vi "Angle_Step.vi"   [LabVIEW 2018]
uses:
  Global/Global Variables/global.vi
  Instrument_Setup.vi
  Global/Global Variables/Data_Display_global.vi
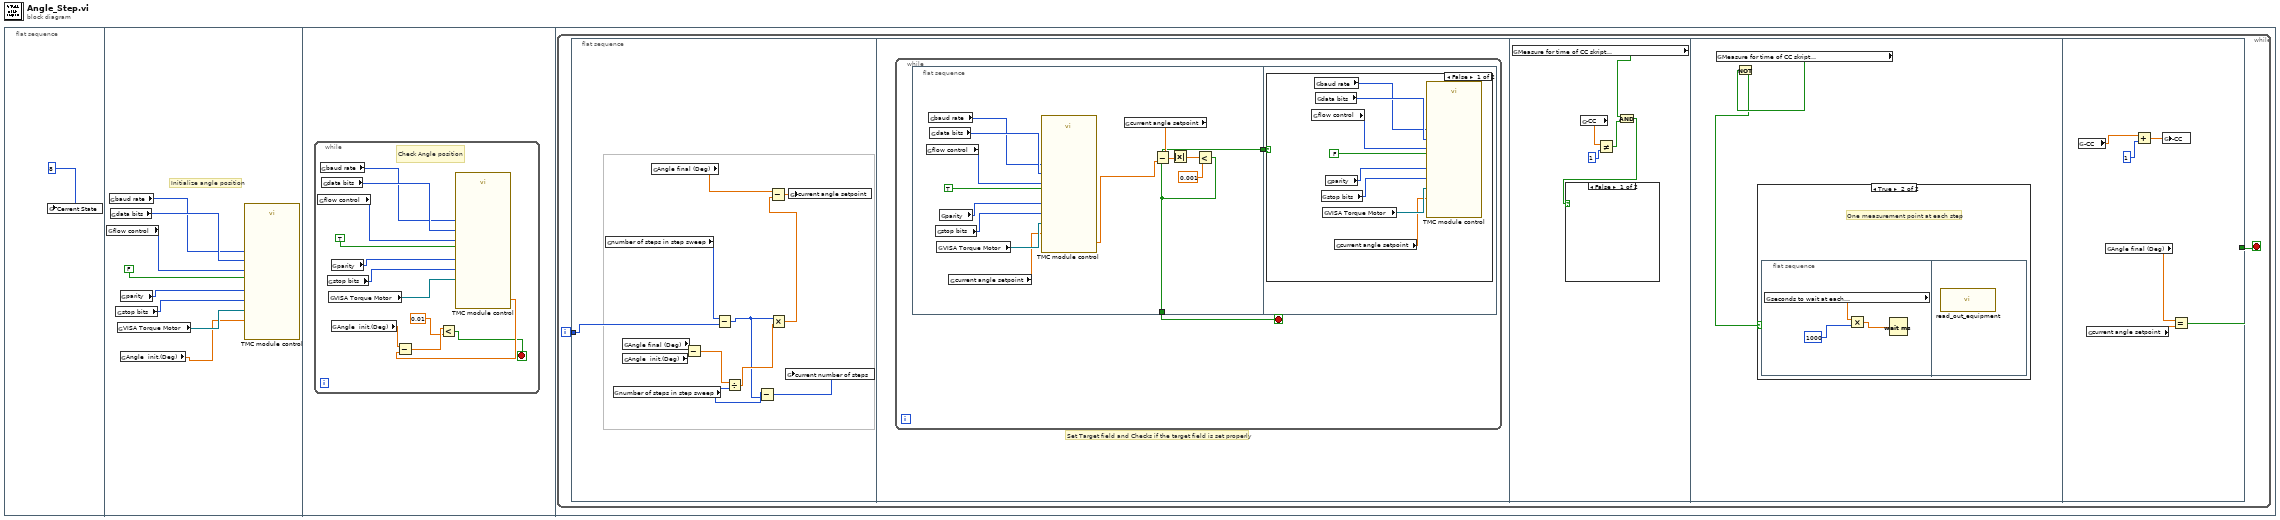
[diagram p0: block diagram]
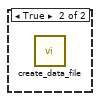
[diagram p3: hidden frame]
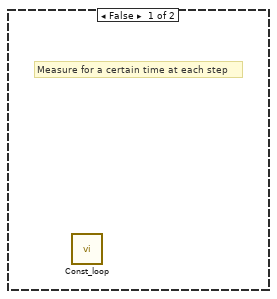
[diagram p4: hidden frame]
diagram:
  n1 = flat-sequence {
    frame #0 {
      n2 = global write "global.vi" "Cerrent State"(8) -> ()
    }
    frame #1 {
      # "Initialize angle position"
      n3 = global read "Instrument_Setup.vi" "flow control"() -> (w9:u16)
      n4 = global read "Instrument_Setup.vi" "baud rate"() -> (w7:u32)
      n5 = global read "Instrument_Setup.vi" "data bits"() -> (w8:u16)
      n6 = global read "Instrument_Setup.vi" "stop bits"() -> (w5:u16)
      n7 = global read "Instrument_Setup.vi" "VISA Torque Motor"() -> (w3:refnum<visa-resource-name>)
      n8 = global read "Instrument_Setup.vi" "parity"() -> (w6:u16)
      n9 = global read "global.vi" "Angle  init.(Deg)"() -> (w2:dbl)
      n10 = call "TMC module control.vi"("Nur Position auslesen"=FALSE, "Winkel [°]"=w2, "flow control"=w9, "VISA resource name"=w3, "stop bits"=w5, "parity"=w6, "data bits"=w8, "baud rate"=w7) -> ()  [unwired: 2 out]
    }
    frame #2 {
      n11 = while {
        stop <- w10 stop-if-true
        # "Check Angle position"
        n12 = global read "Instrument_Setup.vi" "flow control"() -> (w21:u16)
        n13 = global read "Instrument_Setup.vi" "baud rate"() -> (w19:u32)
        n14 = global read "Instrument_Setup.vi" "data bits"() -> (w20:u16)
        n15 = global read "Instrument_Setup.vi" "stop bits"() -> (w17:u16)
        n16 = global read "Instrument_Setup.vi" "VISA Torque Motor"() -> (w15:refnum<visa-resource-name>)
        n17 = global read "Instrument_Setup.vi" "parity"() -> (w18:u16)
        n18 = global read "global.vi" "Angle  init.(Deg)"() -> (w14:dbl)
        n19 = call "TMC module control.vi"("Nur Position auslesen"=TRUE, "flow control"=w21, "VISA resource name"=w15, "stop bits"=w17, "parity"=w18, "data bits"=w20, "baud rate"=w19) -> ("Ausgelesener Winkel [°]"=w13:dbl)  [unwired: 1 in, 1 out]
        n20 = Subtract(x=w14, y=w13) -> (x-y=w12:dbl)
        n21 = Less?(x=w12, y=0.01) -> (x < y?=w10:bool)
      }
    }
    frame #3 {
      n22 = while {
        i -> [w22]
        stop <- w23 stop-if-true
        n23 = flat-sequence {
          tunnel: w22 -> [w24]
          tunnel: [w75] -> w23
          frame #0 {
            n24 = global read "global.vi" "number of steps in step sweep"() -> (w31:i32)
            n25 = global read "global.vi" "number of steps in step sweep"() -> (w29:i32)
            n26 = global read "global.vi" "Angle final (Deg)"() -> (w27:dbl)
            n27 = global read "global.vi" "Angle  init.(Deg)"() -> (w26:dbl)
            n28 = global read "global.vi" "Angle final (Deg)"() -> (w35:dbl)
            n29 = Subtract(x=w27, y=w26) -> (x-y=w25:dbl)
            n30 = Subtract(x=w31, y=w24) -> (x-y=w28:i32)
            n31 = Divide(x=w25, y=w29) -> (x/y=w33:dbl)
            n32 = Subtract(x=w29, y=w28) -> (x-y=w30:i32)
            n33 = Multiply(x=w28, y=w33) -> (x*y=w34:dbl)
            n34 = Subtract(x=w35, y=w34) -> (x-y=w32:dbl)
            n35 = global write "Data_Display_global.vi" "current number of steps"(w30) -> ()
            n36 = global write "Data_Display_global.vi" "current angle setpoint"(w32) -> ()
          }
          frame #1 {
            # "Set Target field and Checks if the target field is set properly"
            n37 = while {
              stop <- w36 stop-if-true
              n38 = flat-sequence {
                tunnel: [w47] -> w37
                tunnel: [w47] -> w36
                tunnel: w37 -> [w52]
                frame #0 {
                  n39 = global read "Instrument_Setup.vi" "flow control"() -> (w45:u16)
                  n40 = global read "Instrument_Setup.vi" "baud rate"() -> (w43:u32)
                  n41 = global read "Instrument_Setup.vi" "data bits"() -> (w44:u16)
                  n42 = global read "Instrument_Setup.vi" "stop bits"() -> (w41:u16)
                  n43 = global read "Instrument_Setup.vi" "VISA Torque Motor"() -> (w39:refnum<visa-resource-name>)
                  n44 = global read "Instrument_Setup.vi" "parity"() -> (w42:u16)
                  n45 = global read "Data_Display_global.vi" "current angle setpoint"() -> (w38:dbl)
                  n46 = call "TMC module control.vi"("Nur Position auslesen"=TRUE, "Winkel [°]"=w38, "flow control"=w45, "VISA resource name"=w39, "stop bits"=w41, "parity"=w42, "data bits"=w44, "baud rate"=w43) -> ("Ausgelesener Winkel [°]"=w46:dbl)  [unwired: 1 out]
                  n47 = global read "Data_Display_global.vi" "current angle setpoint"() -> (w48:dbl)
                  n48 = Subtract(x=w48, y=w46) -> (x-y=w50:dbl)
                  n49 = Absolute Value(x=w50) -> (abs(x)=w49:dbl)
                  n50 = Less?(x=w49, y=0.001) -> (x < y?=w47:bool)
                }
                frame #1 {
                  n51 = case shown="False" w52 {
                    frame False {
                      n52 = global read "Instrument_Setup.vi" "flow control"() -> (w60:u16)
                      n53 = global read "Instrument_Setup.vi" "baud rate"() -> (w58:u32)
                      n54 = global read "Instrument_Setup.vi" "data bits"() -> (w59:u16)
                      n55 = global read "Instrument_Setup.vi" "stop bits"() -> (w56:u16)
                      n56 = global read "Instrument_Setup.vi" "VISA Torque Motor"() -> (w54:refnum<visa-resource-name>)
                      n57 = global read "Instrument_Setup.vi" "parity"() -> (w57:u16)
                      n58 = global read "Data_Display_global.vi" "current angle setpoint"() -> (w53:dbl)
                      n59 = call "TMC module control.vi"("Nur Position auslesen"=FALSE, "Winkel [°]"=w53, "flow control"=w60, "VISA resource name"=w54, "stop bits"=w56, "parity"=w57, "data bits"=w59, "baud rate"=w58) -> ()  [unwired: 2 out]
                    }
                    frame True {
                    }
                  }
                }
              }
            }
          }
          frame #2 {
            n60 = global read "Instrument_Setup.vi" "Measure for time of CC skript\nat each field step point"() -> (w63:bool)
            n61 = global read "global.vi" "-CC"() -> (w65:dbl)
            n62 = Not Equal?(x=w65, y=1) -> (x != y?=w62:bool)
            n63 = And(x=w63, y=w62) -> (x .and. y?=w61:bool)
            n64 = case shown="False" w61 {
              frame False {
              }
              frame True {
                n65 = call "create_data_file.vi"() -> ()  [unwired: 3 in]
              }
            }
          }
          frame #3 {
            n66 = global read "Instrument_Setup.vi" "Measure for time of CC skript\nat each field step point"() -> (w67:bool)
            n67 = Not(x=w67) -> (.not. x?=w66:bool)
            n68 = case shown="True" w66 {
              frame False {
                # "Measure for a certain time at each step"
                n69 = call "Const_loop.vi"() -> ()  [unwired: 4 in]
              }
              frame True {
                # "One measurement point at each step"
                n70 = flat-sequence {
                  frame #0 {
                    n71 = global read "Instrument_Setup.vi" "seconds to wait at each\nfield step in a step sweep"() -> (w70:dbl)
                    n72 = Multiply(x=w70, y=u32 1000 ("milliseconds to wait")) -> (x*y=w68:dbl)
                    n73 = Wait (ms)(milliseconds to wait=w68) -> ()  [unwired: 1 out]
                  }
                  frame #1 {
                    n74 = call "read_out_equipment.vi"() -> ()  [unwired: 1 in]
                  }
                }
              }
            }
          }
          frame #4 {
            n75 = global read "global.vi" "-CC"() -> (w73:dbl)
            n76 = global read "Data_Display_global.vi" "current angle setpoint"() -> (w74:dbl)
            n77 = global read "global.vi" "Angle final (Deg)"() -> (w76:dbl)
            n78 = Add(x=w73, y=1) -> (x+y=w71:dbl)
            n79 = global write "global.vi" "-CC"(w71) -> ()
            n80 = Equal?(x=w76, y=w74) -> (x = y?=w75:bool)
          }
        }
      }
    }
  }
